vi "Get Grid.vi"(8 "error in (no error)":errorcluster, 11 "Cell Context in":refnum<class "Cell Context.lvclass">) -> (0 "error out":errorcluster, 2 "Grid":refnum<k24>, 3 "Cell Context out":refnum<class "Cell Context.lvclass">)   [LabVIEW 2024, in "SourceGrid.lvlib" / "Cell Context.lvclass"]
uses:
  Cell Context.lvclass
  Cell Context.lvclass/Cell Context.ctl
  D:/git/Sourcegrid-LabVIEW/dll/SourceGrid.dll
  dll/SourceGrid.dll
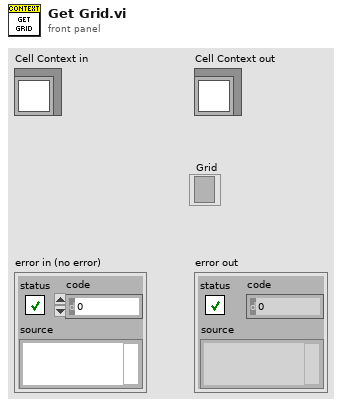
[diagram p1: front panel]
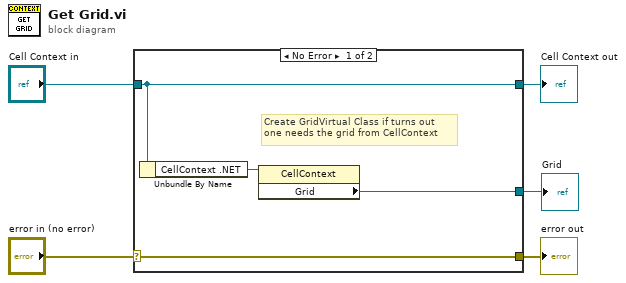
[diagram p0: block diagram]
diagram:
  n1 = case shown="No Error" "error in (no error)" {
    selector: "error in (no error)" -> [w9 w10]
    tunnel: [w9 w10] -> w4
    tunnel: [w8 w11] -> w2
    tunnel: "Cell Context in" -> [w8 w11]
    tunnel: [w6 _] -> w1
    frame No Error {
      # "Create GridVirtual Class if turns out\none needs the grid from CellContext"
      n2 = Unbundle By Name(w8) -> ("CellContext .NET"=w7:refnum<k24>)
      n3 = property class="CellContext"(reference=w7) -> ("Grid"=w6:refnum<k24>)  [unwired: 1 in, 2 out]
    }
    frame Error {
    }
  }
  "error out" <- w4
  "Cell Context out" <- w2
  "Grid" <- w1
